vi "Process Image for Target.vi"(0 "Src Image":T2, 1 "Color Mode":u16(ring)=2 items=["RGB", "HSL", "HSV", "HSI"], 9 "Color Components":T3={"Hue"={110.0, 142.0}, "Sat"={138.0, 255.0}, "Val"={139.0, 198.0}} {"Val" scale=0.0..255.0; "Sat" scale=0.0..255.0; "Hue" scale=0.0..255.0 scale format="%#_3g"}, 11 "Area Cutoff %":dbl=0.05) -> (4 "Src Image Out":T2, 8 "Threshold":T2, 12 "x = y?":cluster{bool, bool, bool, bool}, 13 "Particles gimbal":i32, 14 "area":i32, 15 "Particles":T1(array[cluster]))   [LabVIEW 2013]
doc: "Use color, rectangularity, and aspect ratio to identify and describe potential strips of retroreflective material within the image."
uses:
  <vilib>/vision/Image Controls.llb/IMAQ Image.ctl
  <vilib>/vision/NI_Vision_Development_Module.lvlib
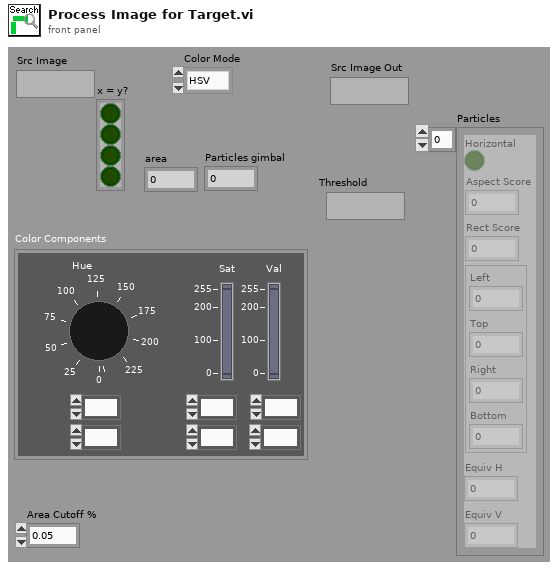
[diagram p1: front panel]
types:
  T1 = cluster{"Horizontal":bool, "Aspect Score":dbl, "Rect Score":dbl, cluster{"Left":dbl, "Top":dbl, "Right":dbl, "Bottom":dbl}, "Equiv H":dbl, "Equiv V":dbl}[]
  T2 = typedef "IMAQ Image.ctl" = refnum<image>
  T3 = cluster{"Hue":cluster{dbl, dbl}, "Sat":cluster{dbl, dbl}, "Val":cluster{dbl, dbl}}
  T4 = typedef "Particle Parameters" = i32
  T5 = typedef "Image Type" = u32
  T6 = cluster{"Pixel Area":dbl, "Rectangle":cluster{"Left":i32, "Top":i32, "Right":i32, "Bottom":i32}}[]
  T7 = cluster{"Numeric":dbl, "Numeric":dbl, "Numeric":dbl, "Numeric":dbl}
  T8 = cluster{"Horizontal":bool, "Score":dbl, "Score":dbl, cluster{"Numeric":dbl, "Numeric":dbl, "Numeric":dbl, "Numeric":dbl}, "Numeric":dbl, "Numeric":dbl}
  T9 = cluster{"Pixel Area":dbl, "Rectangle":cluster{"Left":i32, "Top":i32, "Right":i32, "Bottom":i32}}
  T10 = cluster{"Left":i32, "Top":i32, "Right":i32, "Bottom":i32}
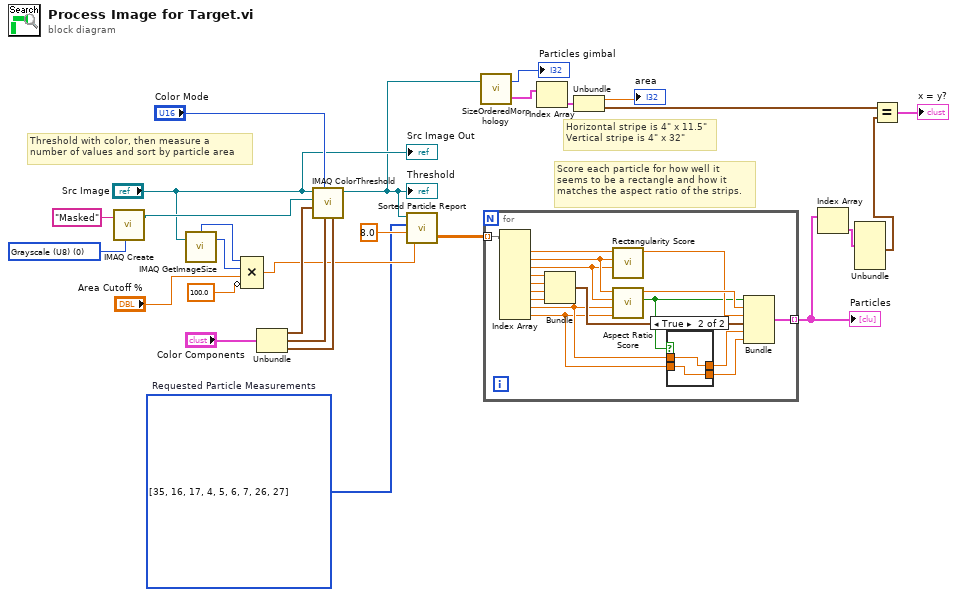
[diagram p0: block diagram]
diagram:
  w13 = T4[] [35, 16, 17, 4, 5, 6, 7, 26, 27] items=["Center of Mass X", "Center of Mass Y", "First Pixel X", "First Pixel Y", "Bounding Rect Left", "Bounding Rect Top", "Bounding Rect Right", "Bounding Rect Bottom", "Max Feret Diameter Start X", "Max Feret Diameter Start Y", "Max Feret Diameter End X", "Max Feret Diameter End Y", "Max Horiz. Segment Length Left", "Max Horiz. Segment Length Right", "Max Horiz. Segment Length Row", "-", "Bounding Rect Width", "Bounding Rect Height", "Bounding Rect Diagonal", "Perimeter", "Convex Hull Perimeter", "Holes' Perimeter", "Max Feret Diameter", "Equivalent Ellipse Major Axis", "Equivalent Ellipse Minor Axis", "Equivalent Ellipse Minor Axis (Feret)", "Equivalent Rect Long Side", "Equivalent Rect Short Side", "Equivalent Rect Diagonal", "Equivalent Rect Short Side (Feret)", "Average Horiz. Segment Length", "Average Vert. Segment Length", "Hydraulic Radius", "Waddel Disk Diameter", "-", "Area", "Holes' Area", "Particle & Holes' Area", "Convex Hull Area", "Image Area", "-", "Number of Holes", "Number of Horiz. Segments", "Number of Vert. Segments", "-", "Orientation", "Max Feret Diameter Orientation", "-", "% Area/Image Area", "% Area/(Particle & Holes' Area)", "Ratio of Equivalent Ellipse Axes", "Ratio of Equivalent Rect Sides", "-", "Elongation Factor", "Compactness Factor", "Heywood Circularity Factor", "Type Factor", "-", "Sum X", "Sum Y", "Sum XX", "Sum XY", "Sum YY", "Sum XXX", "Sum XXY", "Sum XYY", "Sum YYY", "-", "Moment of Inertia XX", "Moment of Inertia XY", "Moment of Inertia YY", "Moment of Inertia XXX", "Moment of Inertia XXY", "Moment of Inertia XYY", "Moment of Inertia YYY", "Norm. Moment of Inertia XX", "Norm. Moment of Inertia XY", "Norm. Moment of Inertia YY", "Norm. Moment of Inertia XXX", "Norm. Moment of Inertia XXY", "Norm. Moment of Inertia XYY", "Norm. Moment of Inertia YYY", "Hu Moment 1", "Hu Moment 2", "Hu Moment 3", "Hu Moment 4", "Hu Moment 5", "Hu Moment 6", "Hu Moment 7"]  # Requested Particle Measurements
  w22 = T5 0 items=["Grayscale (U8)", "Grayscale (I16)", "Grayscale (SGL)", "Complex (CSG)", "RGB (U32)", "HSL (U32)", "RGB (U64)", "Grayscale (U16)"] ("Image Type")
  # "Score each particle for how well it\nseems to be a rectangle and how it\nmatches the aspect ratio of the strips."
  # "Horizontal stripe is 4\" x 11.5\"\nVertical stripe is 4\" x 32\""
  # "Threshold with color, then measure a\nnumber of values and sort by particle area"
  n1 = call "IMAQ Create"("Image Name"="Masked", "Image Type"=w22) -> ("New Image"=w20:T2)  [unwired: 3 in, 1 out]
  n2 = call "IMAQ GetImageSize"("Image"="Src Image") -> ("Y Resolution"=w17:i32, "X Resolution"=w18:i32)  [unwired: 3 in, 1 out]
  n3 = Compound Arithmetic op=MULTIPLY(w18, w17, "Area Cutoff %", invert 100.0 ("value")) -> (w15:dbl)
  n4 = Unbundle("Color Components") -> ("Hue"=w24:cluster{dbl, dbl}, "Sat"=w25:cluster{dbl, dbl}, "Val"=w26:cluster{dbl, dbl})
  n5 = call "IMAQ ColorThreshold"("Blue or Luma or Val or Inten Range"=w26, "Green or Sat Range"=w25, "Color Mode"="Color Mode", "Red or Hue Range"=w24, "Image Dst"=w20, "Image Src"="Src Image") -> ("Image Dst Out"=w10:T2)  [unwired: 4 in, 1 out]
  "Threshold" <- w10
  n6 = call "Sorted Particle Report.vi"("Area Size Limit"=w15, "Particle Count Limit"=8.0, "Pixel Measurements"=w13, "Image in"=w10) -> ("Sorted Data"=w12:dbl[][])  [unwired: 1 out]
  n7 = call "SizeOrderedMorphology.vi"("Image Dst Out"=w10) -> (0:"Particles"=w8:T6, 1:"Particles"=→"Particles gimbal":i32)  [unwired: 1 in]
  n8 = for {
    tunnel: w12 -> [w30] mode=indexing
    tunnel: [w38] -> w3 mode=indexing
    n9 = Index Array(array=w30) -> (element #1=w31:dbl, element #2=w29:dbl, element #3=w28:dbl, element #4=w44:dbl, element #5=w43:dbl, element #6=w42:dbl, element #7=w41:dbl, element #8=w33:dbl, element #9=w32:dbl)  [unwired: 9 in]
    n10 = Bundle("Numeric"=w44, "Numeric"=w43, "Numeric"=w42, "Numeric"=w41) -> (w37:T7)  [unwired: 1 out]
    n11 = call "Rectangularity Score.vi"("Height"=w28, "Width"=w29, "Area"=w31) -> ("Score"=w39:dbl)  [unwired: 8 in]
    n12 = call "Aspect Ratio Score.vi"("Equivalent Rect Short"=w32, "Equivalent Rect Long"=w33, "Height"=w28, "Width"=w29) -> ("Horizontal"=w34:bool, "Score"=w40:dbl)  [unwired: 6 in]
    n13 = case shown="True" w34 {
      tunnel: w32 -> [w45 w48]
      tunnel: w33 -> [w46 w47]
      tunnel: [w46 w48] -> w36
      tunnel: [w45 w47] -> w35
      frame False {
      }
      frame True {
      }
    }
    n14 = Bundle("Horizontal"=w34, "Score"=w40, "Score"=w39, w37, "Numeric"=w35, "Numeric"=w36) -> (w38:T8)  [unwired: 1 out]
  }
  "Particles" <- w3
  n15 = Index Array(array=w8) -> (element=w7:T9)  [unwired: 1 in]
  n16 = Unbundle(w7) -> ("Pixel Area"=→"area":dbl, "Rectangle"=w5:T10)
  n17 = Index Array(array=w3) -> (element=w4:T8)  [unwired: 1 in]
  n18 = Unbundle(w4) -> (w2:T7)  [unwired: 5 out]
  n19 = Equal?(x=w5, y=w2) -> (x = y?=→"x = y?":cluster{bool, bool, bool, bool})
  "Src Image Out" <- "Src Image"
